vi "ADC_Channels_and_Ranges.vi"(2 "Ch & spans":T1[](array[typedef]) {"low limit (-10V)" format="%.3f"; "high limit (10V)" format="%.3f"}, 3 "error in (no error)":errorcluster) -> (6 "Channel list":string, 7 "Range list":string, 9 "error out":errorcluster)   [LabVIEW 2010]
doc: "Takes AI standard channels and limits inputs and converts them to strings ready for the ADC"
uses:
  Controls/Ch_and_Spans.ctl
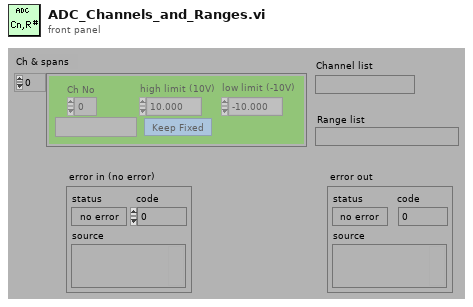
[diagram p1: front panel]
types:
  T1 = typedef "Ch_and_Spans.ctl" = cluster{"high limit (10V)":sgl, "low limit (-10V)":sgl, "Ch No":i16, "Var name":string, "Use Latest Calib":bool}
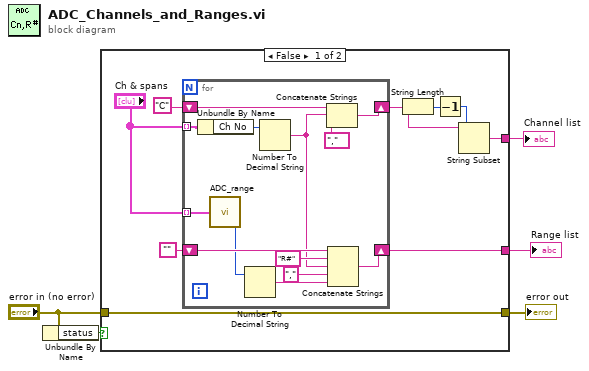
[diagram p0: block diagram]
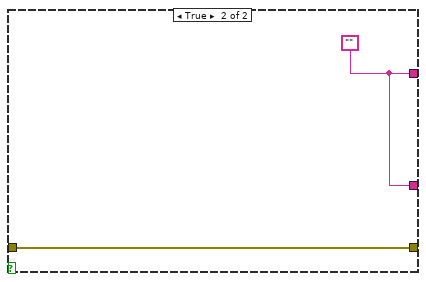
[diagram p2: hidden frame]
diagram:
  n1 = Unbundle By Name("error in (no error)") -> ("status"=w1:bool)
  n2 = case shown="False" w1 {
    tunnel: [w10 w28] -> w4
    tunnel: [w12 w28] -> w5
    tunnel: [w11 w29] -> w3
    tunnel: "error in (no error)" -> [w11 w29]
    frame False {
      n3 = for {
        shift-right: [w22] -> w9
        shift-left: "C" -> [w16]
        shift-right: [w21] -> w12
        shift-left: "" -> [w25]
        tunnel: "Ch & spans" -> [w20] mode=indexing
        tunnel: "Ch & spans" -> [w18] mode=indexing
        n4 = Unbundle By Name(w18) -> ("Ch No"=w17:i16)
        n5 = call "ADC_range.vi"("Channels & Spans"=w20) -> ("Range Code"=w19:i32)  [unwired: 4 out]
        n6 = Number To Decimal String(number=w19) -> (decimal integer string=w24:string)  [unwired: 1 out]
        n7 = Number To Decimal String(number=w17) -> (decimal integer string=w15:string)  [unwired: 1 out]
        n8 = Concatenate Strings(w16, w15, "," ("comma delimiter")) -> (w22:string)
        n9 = Concatenate Strings(w25, "R#", w15, ",", w24) -> (w21:string)
      }
      n10 = String Length(string=w9) -> (length=w8:i32)
      n11 = Decrement(x=w8) -> (x-1=w7:i32)
      n12 = String Subset(string=w9, length (rest)=w7) -> (substring=w10:string)  [unwired: 1 out]
    }
    frame True {
      w28 = ""
    }
  }
  "Range list" <- w5
  "Channel list" <- w4
  "error out" <- w3
